vi "GUI_CH1_Tx.vi"() -> ()   [LabVIEW 2018]
uses:
  Stream/Stream.lvclass
  RxTx/RxTx.lvclass
panel:
  in  "RxTx.lvclass":refnum<class "RxTx.lvclass">
  in  "Stream.lvclass":refnum<class "Stream.lvclass">
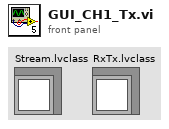
[diagram p1: front panel]
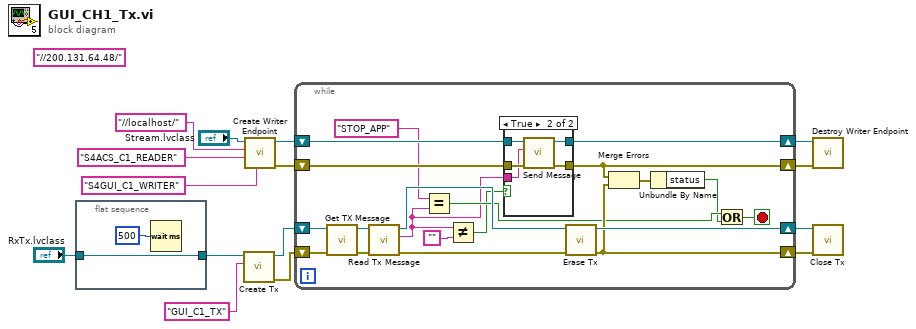
[diagram p0: block diagram]
diagram:
  (unwired) "//200.131.64.48/" ("Reader Name")
  n1 = flat-sequence {
    tunnel: "RxTx.lvclass" -> [w17]
    tunnel: [w17] -> w1
    frame #0 {
      n2 = Wait (ms)(milliseconds to wait=u32 500) -> ()  [unwired: 1 out]
    }
  }
  n3 = call "Create Tx.vi"("Writer Name"="GUI_C1_TX" ("Reader Name"), "RxTx in"=w1) -> ("error out"=w13:errorcluster, "RxTx out"=w14:refnum<class "RxTx.lvclass">)  [unwired: 8 in]
  n4 = call "Create Writer Endpoint.vi"("writer name"="S4GUI_C1_WRITER" ("reader name"), "reader name"="S4ACS_C1_READER", "IP"="//localhost/" ("Reader Name"), "Stream in"="Stream.lvclass") -> ("error out"=w7:errorcluster, "Stream out"=w9:refnum<class "Stream.lvclass">)  [unwired: 6 in]
  n5 = while {
    shift-right: [w29] -> w6
    shift-left: w7 -> [w31]
    shift-right: [w30] -> w15
    shift-left: w9 -> [w32]
    shift-right: [w24] -> w10
    shift-left: w13 -> [w33]
    shift-right: [w26] -> w11
    shift-left: w14 -> [w34]
    stop <- w21 stop-if-true
    n6 = call "Get TX Message.vi"("error in (no error)"=w33, "RxTx in"=w34) -> ("error out"=w36:errorcluster, "RxTx out"=w35:refnum<class "RxTx.lvclass">)  [unwired: 8 in]
    n7 = call "Read Tx Message.vi"("error in (no error)"=w36, "RxTx in"=w35) -> ("error out"=w25:errorcluster, "Tx Message"=w19:string, "RxTx out"=w27:refnum<class "RxTx.lvclass">)  [unwired: 7 in]
    n8 = Equal?(x="STOP_APP", y=w19) -> (x = y?=w23:bool)
    n9 = Not Equal?(x=w19, y="") -> (x != y?=w18:bool)
    n10 = case shown="True" w18 {
      tunnel: w32 -> [w39 w44]
      tunnel: w31 -> [w38 w43]
      tunnel: [w39 w42] -> w30
      tunnel: w19 -> [_ w41]
      tunnel: [w38 w40] -> w29
      frame False {
      }
      frame True {
        n11 = call "Send Message.vi"("error in (no error)"=w43, "Message"=w41, "Stream in"=w44) -> ("error out"=w40:errorcluster, "Stream out"=w42:refnum<class "Stream.lvclass">)  [unwired: 7 in]
      }
    }
    n12 = call "Erase Tx.vi"("error in (no error)"=w25, "RxTx in"=w27) -> ("error out"=w24:errorcluster, "RxTx out"=w26:refnum<class "RxTx.lvclass">)  [unwired: 8 in]
    n13 = Merge Errors(w29, w24) -> (w37:errorcluster)
    n14 = Unbundle By Name(w37) -> ("status"=w22:bool)
    n15 = Or(x=w23, y=w22) -> (x .or. y?=w21:bool)
  }
  n16 = call "Destroy Writer Endpoint.vi"("error in (no error)"=w6, "Stream in"=w15) -> ()  [unwired: 8 in, 2 out]
  n17 = call "Close Tx.vi"("error in (no error)"=w10, "RxTx in"=w11) -> ()  [unwired: 8 in, 2 out]
